vi "Initialize Draw Area State.vi"(11 "DrawAreaSize":T2) -> (3 "draw area state":T1)   [LabVIEW 2017, in "NI_Robotics_Attitude Picture.lvlib"]
uses:
  <vilib>/robotics/Controls/Attitude Indicator/Attitude Picture/NI_Robotics_Attitude Picture.lvlib
  <vilib>/Utility/miscctls.llb/LVBoundsTypeDef.ctl
  <vilib>/robotics/Controls/Attitude Indicator/Attitude Picture/Draw Area State.ctl
  <vilib>/Utility/AngleManip/Degrees to Radians (Scalar DBL).vi
  <vilib>/Utility/AngleManip/NI_AngleManipulation.lvlib
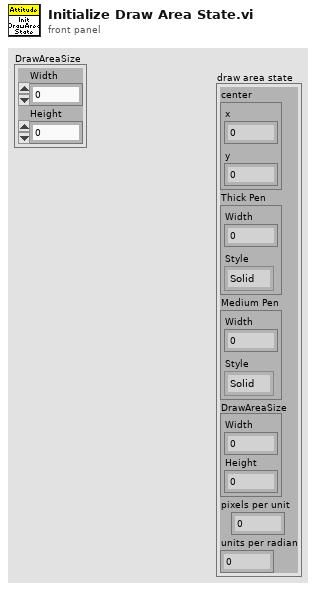
[diagram p1: front panel]
types:
  T1 = typedef "NI_Robotics_Attitude Picture.lvlib/Draw Area State.ctl" = cluster{"center":cluster{"x":i16, "y":i16}, "Thick Pen":cluster{"Width":u16, "Style":enum32{"Solid", "Dash", "Dot", "DashDot", "DashDotDot"}}, "Medium Pen":cluster{"Width":u16, "Style":enum32{"Solid", "Dash", "Dot", "DashDot", "DashDotDot"}}, "DrawAreaSize":T2, "pixels per unit":dbl, "units per radian":dbl}
  T2 = typedef "LVBoundsTypeDef.ctl" = cluster{"Width":u32, "Height":u32}
  T3 = cluster{"Width":u16, "Style":enum32{"Solid", "Dash", "Dot", "DashDot", "DashDotDot"}}
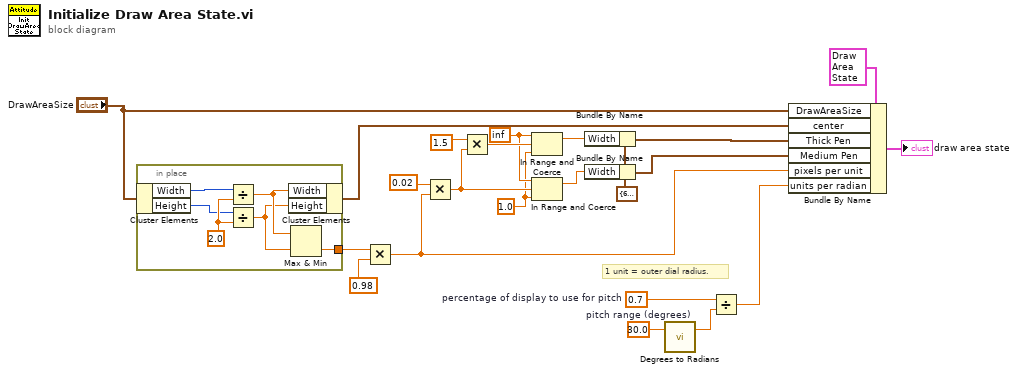
[diagram p0: block diagram]
diagram:
  w4 = 1.0 ("y")
  w5 = inf
  w13 = T3 {"Width"=6, "Style"=enum."Solid"} ("pen")
  w19 = 30.0  # pitch range (degrees)
  w10 = 0.7  # percentage of display to use for pitch
  # "1 unit = outer dial radius."
  n1 = in-place {
    in-place-border: [w25] -> w2
    w28 = 2.0 ("y")
    n2 = in-place-cluster #1("DrawAreaSize") -> ("Width"=w27:u32, "Height"=w26:u32)
    n3 = Divide(x=w27, y=w28) -> (x/y=w24:dbl)
    n4 = Divide(x=w26, y=w28) -> (x/y=w23:dbl)
    n5 = in-place-cluster #1("Width"=w24, "Height"=w23) -> (w20:T2)
    n6 = Max & Min(x=w24, y=w23) -> (min(x,y)=w25:dbl)  [unwired: 1 out]
  }
  n7 = Multiply(x=w2, y=0.98) -> (x*y=w3:dbl)
  n8 = Multiply(x=0.02 ("y"), y=w3) -> (x*y=w7:dbl)
  n9 = Multiply(x=1.5 ("y"), y=w7) -> (x*y=w9:dbl)
  n10 = In Range and Coerce(upper limit=w5, x=w9, lower limit=w4) -> (coerced(x)=w8:dbl)  [unwired: 1 out]
  n11 = In Range and Coerce(upper limit=w5, x=w7, lower limit=w4) -> (coerced(x)=w6:dbl)  [unwired: 1 out]
  n12 = Bundle By Name(cluster=w13, "Width"=w8) -> (w14:T3)
  n13 = Bundle By Name(cluster=w13, "Width"=w6) -> (w12:T3)
  n14 = call-poly <vilib>:"Degrees to Radians.vi"("angle (deg)"=w19) -> ("angle (rad)"=w18:dbl)  [unwired: 2 in]
  n15 = Divide(x=w10, y=w18) -> (x/y=w17:dbl)
  n16 = Bundle By Name(cluster=T1 {"center"={"x"=0, "y"=0}, "Thick Pen"={"Width"=0, "Style"=enum."Solid"}, "Medium Pen"={"Width"=0, "Style"=enum."Solid"}, "DrawAreaSize"={"Width"=0, "Height"=0}, "pixels per unit"=0.0, "units per radian"=0.0} ("draw area state"), "DrawAreaSize"="DrawAreaSize", "center"=w20, "Thick Pen"=w14, "Medium Pen"=w12, "pixels per unit"=w3, "units per radian"=w17) -> (→"draw area state":T1)
